vi "CreateUserEvents.vi"(8 "error in (no error)":errorcluster) -> (0 "error out":errorcluster, 2 "Event Cluster":T1, 3 "Event Registration Refnum out":refnum<event-registration>)   [LabVIEW 2015]
uses:
  controls/UI Events.ctl
  User Events.lvlib
panel:
  in  "Cluster":T2
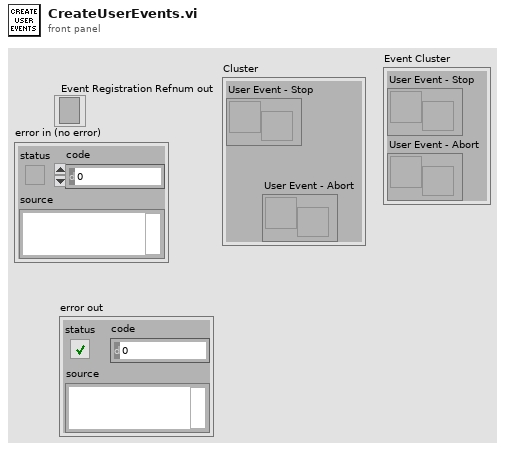
[diagram p1: front panel]
types:
  T1 = typedef "UI Events.ctl" = cluster{"User Event - Stop":refnum<user-event>, "User Event - Abort":refnum<user-event>}
  T2 = cluster{"User Event - Stop":refnum<user-event>, "User Event - Abort":refnum<user-event>}
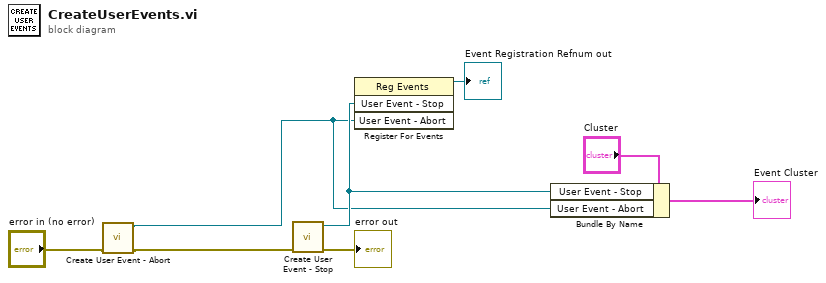
[diagram p0: block diagram]
diagram:
  n1 = call "Create User Event - Abort.vi"("error in (no error)"="error in (no error)") -> ("error out"=w2:errorcluster, "User Event - Abort"=w3:refnum<user-event>)  [unwired: 9 in]
  n2 = call "Create User Event - Stop.vi"("error in (no error)"=w2) -> ("error out"=→"error out":errorcluster, "User Event - Stop"=w6:refnum<user-event>)  [unwired: 9 in]
  n3 = register-events(w6, w3) -> (reference out=→"Event Registration Refnum out":refnum<event-registration>)  [unwired: 2 in, 1 out]
  n4 = Bundle By Name(cluster="Cluster", "User Event - Stop"=w6, "User Event - Abort"=w3) -> (→"Event Cluster":T2)
